vi "Read ADU Packet1.vi"(8 "error in":errorcluster, 10 "isMaster (f)":bool, 11 "ASCII transmission data unit in":refnum<class "ASCII Data Unit.lvclass">) -> (0 "error out":errorcluster, 1 "modbus data unit":refnum<class "Modbus Data Unit.lvclass">, 3 "ASCII transmission data unit out":refnum<class "ASCII Data Unit.lvclass">, 5 "PDU Valid?":bool)   [LabVIEW 2021, in "ASCII Data Unit.lvclass"]
uses:
  ASCII Data Unit.lvclass
  D:/my_projects/projects/Algorithms/Labview/21/Modbus_v121c/Transmission Data Unit/Serial Interface/Serial Data Unit.lvclass
  D:/my_projects/projects/Algorithms/Labview/21/Modbus_v121c/Transmission Data Unit/Transmission Data Unit.lvclass
  Modbus Data Unit/Modbus Data Unit.lvclass
  Transmission Data Unit.lvclass/Transmission Data Unit.ctl
  Serial Interface/Serial Data Unit.lvclass/Serial Data Unit.ctl
  Modbus Data Unit/Modbus Data Unit.lvclass/Modbus Data Unit.ctl
  LRC-8.vi
  <vilib>/ErrorRing/Error Ring.xnode
  Transmission Data Unit.lvclass
  Serial Interface/Serial Data Unit.lvclass
  Network Interface/Serial Interface/Serial Shared Components/Serial Shared Components.lvlib
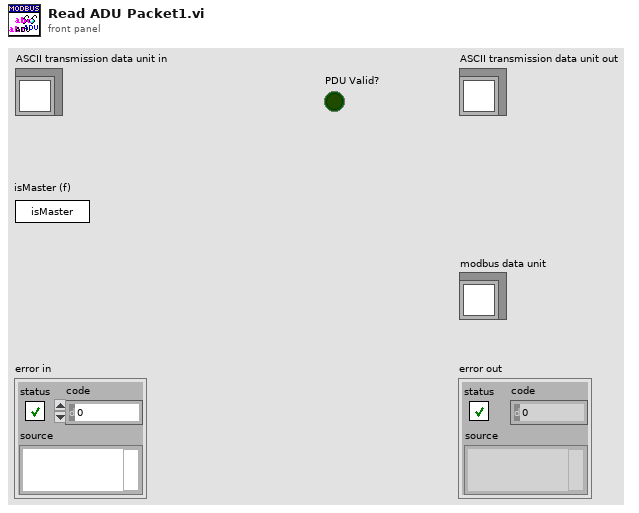
[diagram p1: front panel]
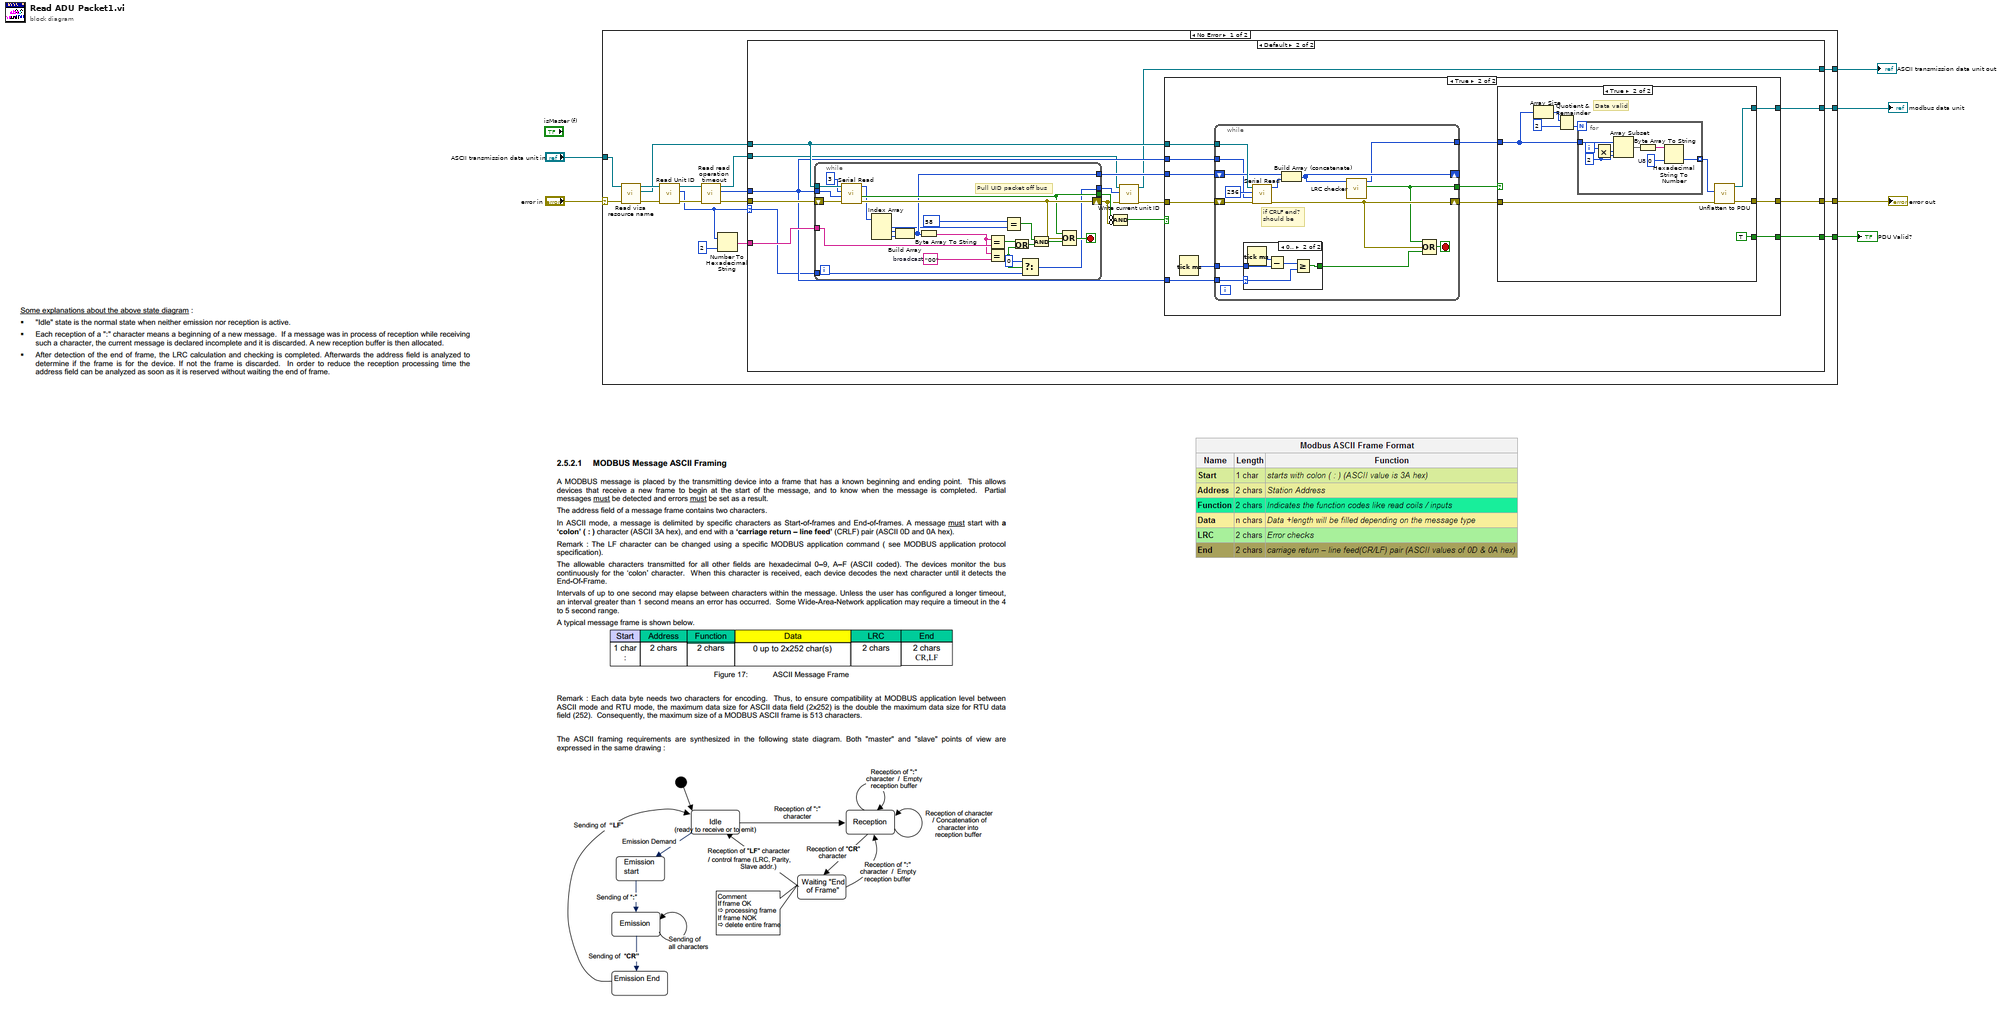
[diagram p0: block diagram]
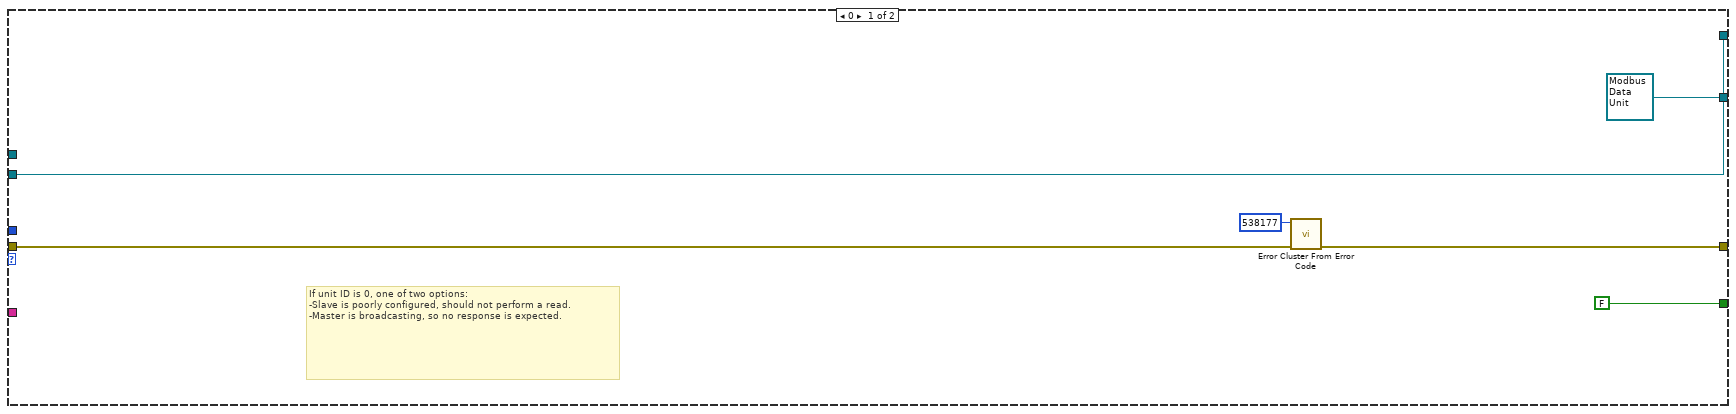
[diagram p2: hidden frame]
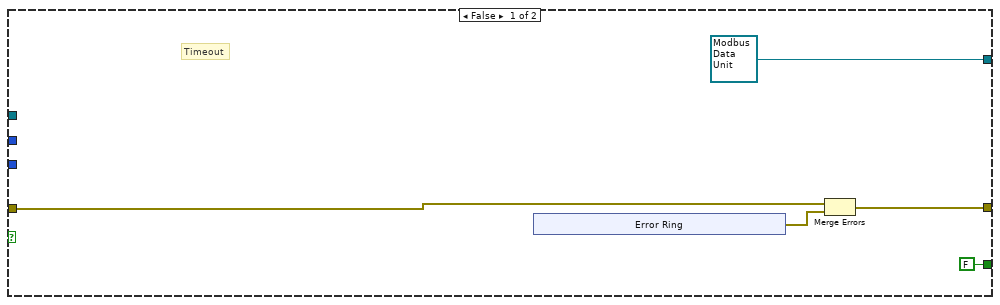
[diagram p3: hidden frame]
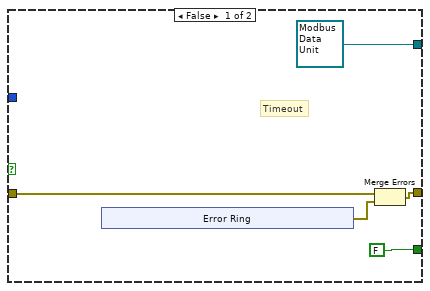
[diagram p4: hidden frame]
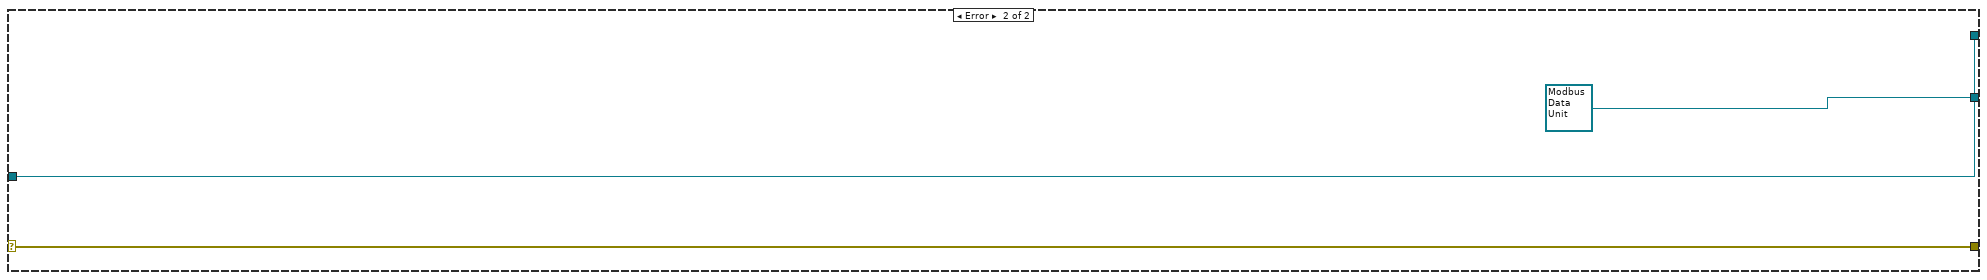
[diagram p6: hidden frame]
diagram:
  n1 = case shown="No Error" "error in" {
    selector: "error in" -> [w11 w138]
    tunnel: [w23 w138] -> w3
    tunnel: "ASCII transmission data unit in" -> [w9 w136]
    tunnel: [w22 refnum<class "Modbus Data Unit.lvclass"> refnum ("modbus data unit")] -> w4
    tunnel: [w17 _] -> w2
    tunnel: [w12 w136] -> w1
    frame No Error {
      n2 = call "Read visa resource name.vi"("error in (no error)"=w11, "Serial Data Unit in"=w9) -> ("error out"=w10:errorcluster, "visa resource name"=w7:refnum<visa-resource-name>, "Serial Data Unit out"=w8:refnum<class "ASCII Data Unit.lvclass">)  [unwired: 7 in]
      n3 = call "Read Unit ID.vi"("error in"=w10, "transmission data unit in"=w8) -> ("error out"=w20:errorcluster, "unit ID"=w15:u8, "transmission data unit out"=w21:refnum<class "ASCII Data Unit.lvclass">)  [unwired: 7 in]
      n4 = call "Read read operation timeout.vi"("error in (no error)"=w20, "transmission data unit in"=w21) -> ("error out"=w19:errorcluster, "read operation timeout"=w18:i32, "transmission data unit out"=w13:refnum<class "ASCII Data Unit.lvclass">)  [unwired: 7 in]
      n5 = Number To Hexadecimal String(1:i16 2 ("width (-)"), 2:w15) -> (0:w14:string)
      n6 = case shown="Default" w15 {
        selector: w15 -> [_ w30]
        tunnel: w19 -> [w29 w42]
        tunnel: [w26 w45] -> w23
        tunnel: [refnum<class "Modbus Data Unit.lvclass"> refnum ("modbus data unit out") w44] -> w22
        tunnel: w7 -> [_ w41]
        tunnel: w18 -> [_ w36]
        tunnel: [FALSE w43] -> w17
        tunnel: w14 -> [_ w40]
        tunnel: w13 -> [w24 w33]
        tunnel: [w24 w31] -> w12
        frame 0 {
          # "If unit ID is 0, one of two options:\n-Slave is poorly configured, should not perform a read.\n-Master is broadcasting, so no response is expected."
          n7 = call <vilib>:"Error Cluster From Error Code.vi"("error in (no error)"=w29, "error code (0)"=538177) -> ("error out"=w26:errorcluster)  [unwired: 7 in]
        }
        frame Default {
          n8 = while {
            shift-right: [w132] -> w35
            shift-left: w42 -> [w135]
            tunnel: w36 -> [w130]
            tunnel: [w128] -> w39
            tunnel: [w121] -> w37
            tunnel: w41 -> [w134]
            tunnel: w40 -> [w122]
            tunnel: [w112] -> w32
            tunnel: w30 -> [w114]
            stop <- w133 stop-if-true
            w117 = "00"  # broadcast
            # "Pull UID packet off bus"
            n9 = call "Serial Read.vi"("error in"=w135, "timeout (ms)"=w130, "bytes to read"=3, "Visa Resource"=w134) -> ("error out"=w132:errorcluster, "timed out?"=w128:bool, "data"=w127:u8[])  [unwired: 5 in]
            n10 = Index Array(array=w127) -> (element #1=w116:u8, element #2=w124:u8, element #3=w123:u8)  [unwired: 3 in]
            n11 = Build Array(w124, w123) -> (w121:u8[])
            n12 = Byte Array To String(unsigned byte array=w121) -> (string=w118:string)
            n13 = Equal?(x=w118, y=w122) -> (x = y?=w119:bool)
            n14 = Equal?(x=w118, y=w117) -> (x = y?=w115:bool)
            n15 = Equal?(x=u8 58 ("y"), y=w116) -> (x = y?=w125:bool)
            n16 = Or(x=w119, y=w115) -> (x .or. y?=w120:bool)
            n17 = Select(t=u8 0, s=w115, f=w114) -> (s? t:f=w112:u8)
            n18 = And(x=w125, y=w120) -> (x .and. y?=w129:bool)
            n19 = Compound Arithmetic op=OR(w128, w132, w129) -> (w133:bool)
          }
          n20 = Compound Arithmetic op=AND(invert w39, invert w35) -> (w38:bool)
          n21 = call "Write current unit ID.vi"("error in"=w35, "request unit ID"=w32, "Serial Data Unit in"=w33) -> ("error out"=w34:errorcluster, "Serial Data Unit out"=w31:refnum<class "ASCII Data Unit.lvclass">)  [unwired: 7 in]
          n22 = case shown="True" w38 {
            tunnel: w34 -> [w48 w66]
            tunnel: [w49 w58] -> w45
            tunnel: [refnum<class "Modbus Data Unit.lvclass"> refnum ("modbus data unit out") w59] -> w44
            tunnel: w41 -> [_ w62]
            tunnel: w37 -> [_ w63]
            tunnel: w36 -> [_ w64]
            tunnel: [FALSE w56] -> w43
            tunnel: w36 -> [_ w55]
            frame False {
              # "Timeout"
              n23 = xnode "Error Ring"() -> ("error out"=w50:errorcluster)
              n24 = Merge Errors(w48, w50) -> (w49:errorcluster)
            }
            frame True {
              n25 = Tick Count (ms)() -> (millisecond timer value=w65:u32)
              n26 = while {
                shift-right: [w98] -> w60
                shift-left: w66 -> [w103]
                tunnel: w65 -> [w106]
                tunnel: w64 -> [w93]
                shift-right: [w97] -> _
                shift-left: w63 -> [w100]
                tunnel: w62 -> [w102]
                tunnel: [w95] -> w61
                tunnel: [w96] -> w57
                tunnel: w55 -> [w94]
                stop <- w105 stop-if-true
                # "if CRLF end?\nshould be"
                n27 = case shown="0.." w93 {
                  selector: w93 -> [_ w107]
                  tunnel: w106 -> [_ w111]
                  tunnel: [_ w108] -> w104
                  frame ..-1 {
                    # "no t/o"
                  }
                  frame 0.. {
                    n28 = Tick Count (ms)() -> (millisecond timer value=w110:u32)
                    n29 = Subtract(x=w110, y=w111) -> (x-y=w109:u32)
                    n30 = Greater Or Equal?(x=w109, y=w107) -> (x >= y?=w108:bool)
                  }
                }
                n31 = call "Serial Read.vi"("error in"=w103, "timeout (ms)"=w94, "bytes to read"=256, "Visa Resource"=w102) -> ("error out"=w98:errorcluster, "data"=w99:u8[])  [unwired: 5 in, 1 out]
                n32 = Build Array (concatenate)(w100, w99) -> (w97:u8[])
                n33 = call "LRC checker.vi"("Data In"=w97) -> ("Valid?"=w95:bool, "Function Data Out"=w96:u8[])  [unwired: 9 in]
                n34 = Compound Arithmetic op=OR(w95, w98, w104) -> (w105:bool)
              }
              n35 = case shown="True" w61 {
                tunnel: w60 -> [w69 w82]
                tunnel: [refnum<class "Modbus Data Unit.lvclass"> refnum ("modbus data unit") w83] -> w59
                tunnel: [w68 w84] -> w58
                tunnel: w57 -> [_ w77]
                tunnel: [FALSE TRUE] -> w56
                frame False {
                  # "Timeout"
                  n36 = xnode "Error Ring"() -> ("error out"=w70:errorcluster)
                  n37 = Merge Errors(w69, w70) -> (w68:errorcluster)
                }
                frame True {
                  # "Data valid"
                  n38 = Array Size(array=w77) -> (size(s)=w81:i32)
                  n39 = Quotient & Remainder(x=w81, y=2) -> (floor(x/y)=w79:i32)  [unwired: 1 out]
                  n40 = for {
                    N: w79 -> [_]
                    tunnel: w77 -> [w92]
                    tunnel: [w85] -> w78 mode=indexing
                    i -> [w91]
                    w86 = u8 0  # U8
                    w90 = 2 ("length")
                    n41 = Multiply(x=w91, y=w90) -> (x*y=w89:i32)
                    n42 = Array Subset(array=w92, index=w89, length=w90) -> (w88:u8[])
                    n43 = Byte Array To String(unsigned byte array=w88) -> (string=w87:string)
                    n44 = Hexadecimal String To Number(string=w87, default (0uL)=w86) -> (number=w85:u8)  [unwired: 2 out]
                  }
                  n45 = call "Unflatten to PDU.vi"("error in"=w82, "modbus data unit data"=w78) -> ("error out"=w84:errorcluster, "modbus data unit out"=w83:refnum<class "Modbus Data Unit.lvclass">)  [unwired: 8 in]
                }
              }
            }
          }
        }
      }
    }
    frame Error {
    }
  }
  "ASCII transmission data unit out" <- w1
  "modbus data unit" <- w4
  "error out" <- w3
  "PDU Valid?" <- w2
